vi "ranking labview.vi"() -> ()   [LabVIEW 2015]
panel:
  out "Array":T1(array[cluster])
  out "EXAM 2 SCORES":dbl[](array[numeric])
  in  "Number of students":dbl
  out "EXAM 1 SCORES":dbl[](array[numeric])
  out "EXAM 3 SCORES":dbl[](array[numeric])
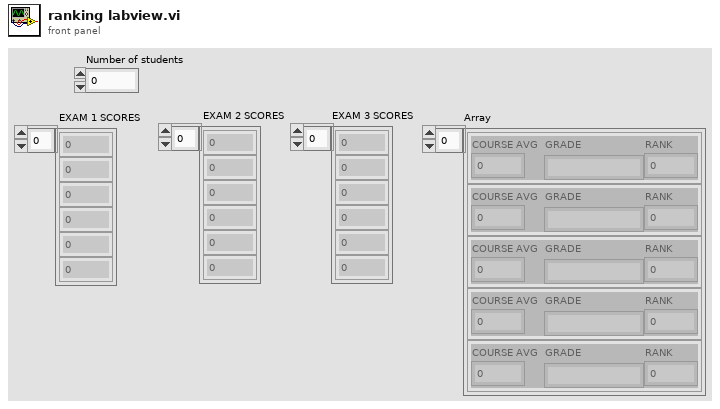
[diagram p1: front panel]
types:
  T1 = cluster{"COURSE AVG":dbl, "GRADE":string, "RANK":dbl}[]
  T2 = cluster{"COURSE AVG":dbl, "GRADE":string, "RANK":dbl}
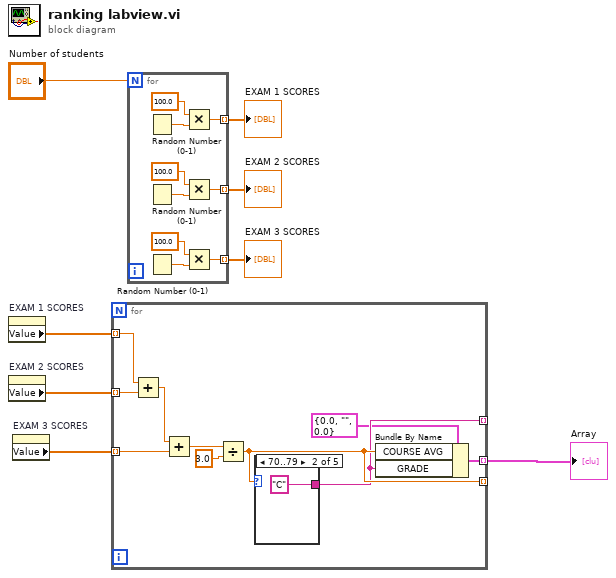
[diagram p0: block diagram]
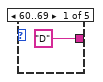
[diagram p2: hidden frame]
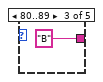
[diagram p3: hidden frame]
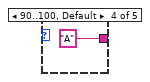
[diagram p4: hidden frame]
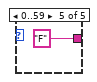
[diagram p5: hidden frame]
diagram:
  n1 = property on="EXAM 1 SCORES" class="Arr (strict)"() -> ("Value"=w5:dbl[])  [unwired: 2 in, 2 out]
  n2 = property on="EXAM 2 SCORES" class="Arr (strict)"() -> ("Value"=w4:dbl[])  [unwired: 2 in, 2 out]
  n3 = property on="EXAM 3 SCORES" class="Arr (strict)"() -> ("Value"=w3:dbl[])  [unwired: 2 in, 2 out]
  n4 = for {
    tunnel: w5 -> [w18] mode=indexing
    tunnel: w4 -> [w17] mode=indexing
    tunnel: w3 -> [w15] mode=indexing
    tunnel: [w12] -> _ mode=indexing
    tunnel: [w11] -> _ mode=indexing
    tunnel: [w9] -> w1 mode=indexing
    n5 = Add(x=w18, y=w17) -> (x+y=w16:dbl)
    n6 = Add(x=w16, y=w15) -> (x+y=w14:dbl)
    n7 = Divide(x=w14, y=3.0) -> (x/y=w12:dbl)
    n8 = case shown="70..79" w12 {
      tunnel: ["D" "C" "B" "A" "F"] -> w11
      frame 60..69 {
      }
      frame 70..79 {
      }
      frame 80..89 {
      }
      frame 90..100, Default {
      }
      frame 0..59 {
      }
    }
    n9 = Bundle By Name(cluster=T2 {"COURSE AVG"=0.0, "GRADE"="", "RANK"=0.0} ("Cluster"), "COURSE AVG"=w12, "GRADE"=w11) -> (w9:T2)
  }
  "Array" <- w1
  n10 = for {
    N: "Number of students" -> [_]
    tunnel: [w26] -> w6 mode=indexing
    tunnel: [w25] -> w8 mode=indexing
    tunnel: [w24] -> w7 mode=indexing
    n11 = Random Number (0-1)() -> (number: 0 to 1=w27:dbl)
    n12 = Random Number (0-1)() -> (number: 0 to 1=w28:dbl)
    n13 = Random Number (0-1)() -> (number: 0 to 1=w29:dbl)
    n14 = Multiply(x=100.0, y=w27) -> (x*y=w24:dbl)
    n15 = Multiply(x=100.0, y=w28) -> (x*y=w26:dbl)
    n16 = Multiply(x=100.0, y=w29) -> (x*y=w25:dbl)
  }
  "EXAM 3 SCORES" <- w8
  "EXAM 1 SCORES" <- w7
  "EXAM 2 SCORES" <- w6
